vi "构建程序框图.vi"() -> ()   [LabVIEW 2010]
uses:
  <vilib>/Analysis/NI_AALBase.lvlib
panel:
  in  "stop":bool
  out "平均值":dbl
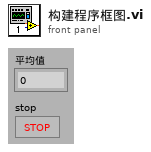
[diagram p1: front panel]
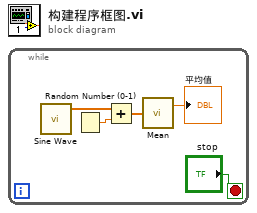
[diagram p0: block diagram]
diagram:
  n1 = while {
    stop <- "stop" stop-if-true
    n2 = call <vilib>:"Sine Wave.vi"() -> ("sine wave"=w5:dbl[])  [unwired: 5 in, 2 out]
    n3 = Random Number (0-1)() -> (number: 0 to 1=w4:dbl)
    n4 = Add(x=w5, y=w4) -> (x+y=w3:dbl[])
    n5 = call <vilib>:"Mean.vi"("X"=w3) -> ("mean"=→"平均值":dbl)  [unwired: 1 out]
  }
